vi "ExDataCollectFocus2StripROT.vi"() -> ()   [LabVIEW 2010]
uses:
  Open-Close Hardware/CamHandle.vi
panel:
  out "vert shift time":dbl format="%.2f"
  out "horz shift time":dbl format="%.2f"
  out "Read Out":dbl format="%.2f"
  out "Strip 2":u16[](graph)
  out "Strip":u16[](graph)
  in  "Stop collection":bool
  out "ready to \nstart":bool
  in  "Start collection":bool
  in  "Exposure":dbl min=0.0 step=0.001 format="%.3f"
  out "error out":errorcluster
  in  "error in (no error)":errorcluster
  # "ExDataCollect2StripROT:\nthis example collects data for 2 strips.\nIt also displays the Read Out time, horizontal shift time, and vertical shift time.\nRun this vi and wait for the ready to start to turn green.\nThen hit the start button to collect and display the strips as graphs"
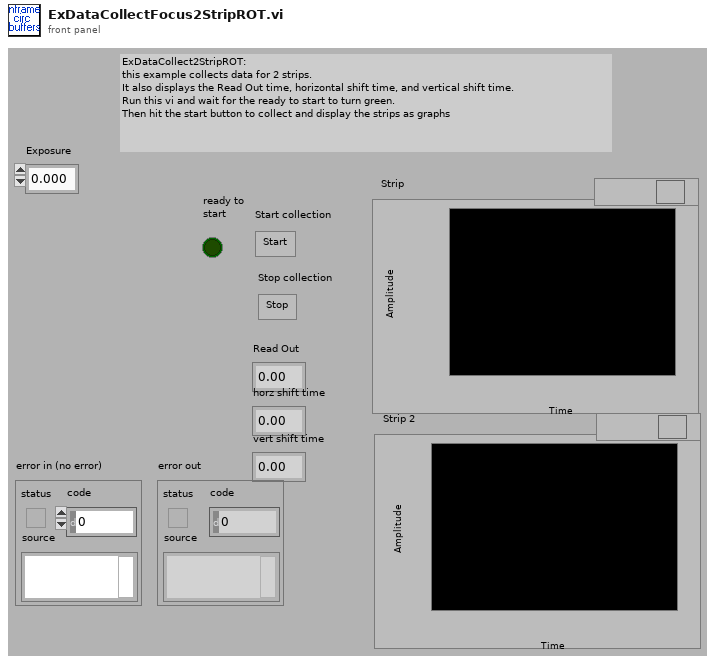
[diagram p1: front panel]
types:
  T1 = cluster{"acquire focus mode":u32, "Exposure":dbl, i32, "Software accumulation":u32}
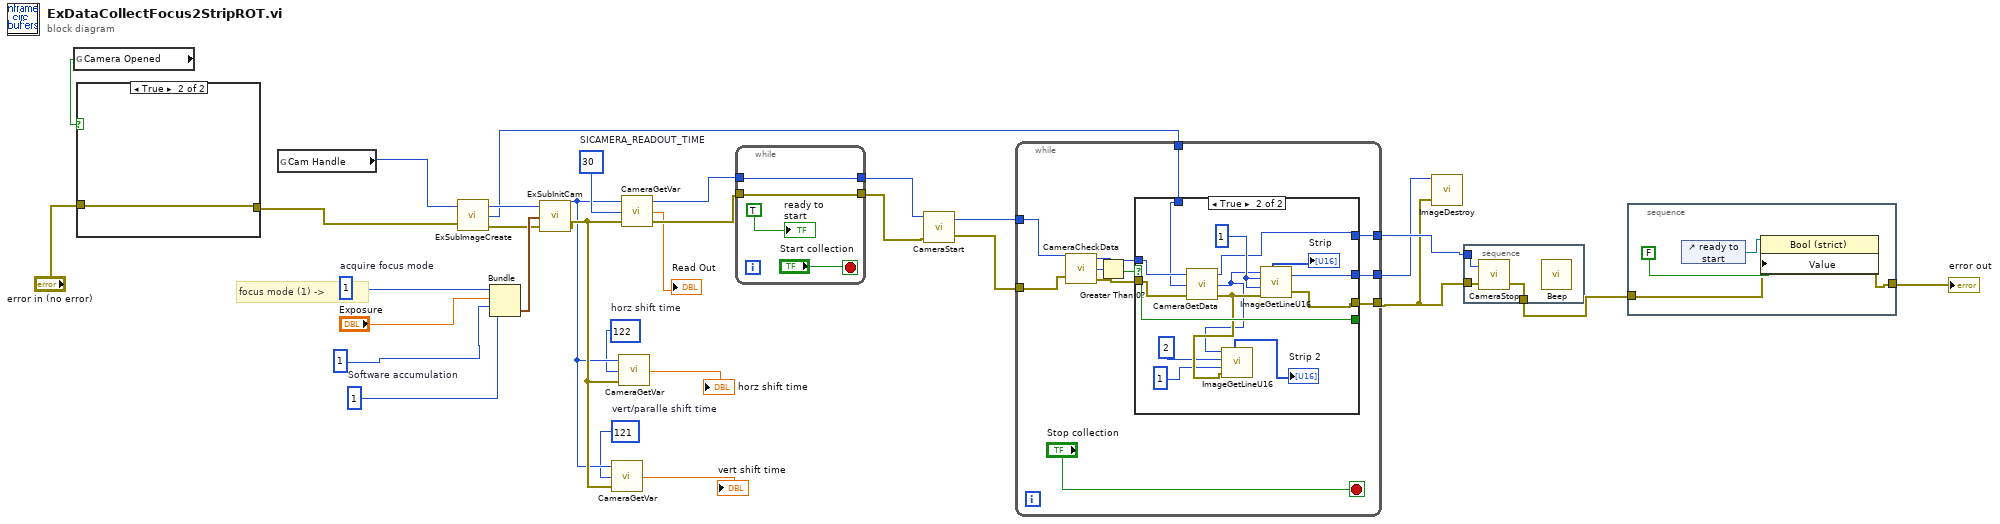
[diagram p0: block diagram]
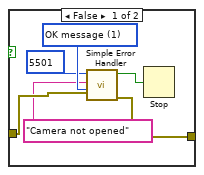
[diagram p3: hidden frame]
diagram:
  w2 = 122  # horz shift time
  w3 = 121  # vert/paralle shift time
  w8 = 30  # SICAMERA_READOUT_TIME
  w29 = u32 1  # acquire focus mode
  w28 = u32 1  # Software accumulation
  # "focus mode (1) ->"
  n1 = global read "CamHandle.vi" "Camera Opened"() -> (w26:bool)
  n2 = case shown="True" w26 {
    tunnel: "error in (no error)" -> [w36 w38]
    tunnel: [w35 w38] -> w18
    frame False {
      w37 = u16 1 items=["no dialog", "OK message", "continue or stop message"] ("type of dialog (OK msg:1)")
      n3 = call <vilib>:"Simple Error Handler.vi"("error code (no error:0)"=5501, "error source (\" \")"="Camera not opened", "type of dialog (OK msg:1)"=w37, "error in (no error)"=w36) -> ("error?"=w33:bool, "error out"=w35:errorcluster)  [unwired: 1 in, 3 out]
      n4 = Stop(stop? (T)=w33) -> ()
    }
    frame True {
    }
  }
  n5 = global read "CamHandle.vi" "Cam Handle"() -> (w20:u32)
  n6 = call "ExSubImageCreate.vi"("Camera Handle"=w20, "error in (no error)"=w18) -> ("Camera Handle"=w19:u32, "Data Handle"=w16:u32, "error out"=w17:errorcluster)
  n7 = Bundle("acquire focus mode"=w29, "Exposure"="Exposure", 1, "Software accumulation"=w28) -> (w30:T1)  [unwired: 1 in]
  n8 = call "ExSubInitCam.vi"("error in (no error)"=w17, "Camera Information"=w30, "Camera Handle"=w19) -> ("error out"=w7:errorcluster, "Camera Handle"=w4:u32)
  n9 = call <userlib>:"CameraGetVar.vi"("error in"=w7, "Parameter ID"=w3, "Camera Handle"=w4) -> ("Value"=→"vert shift time":dbl)  [unwired: 2 out]
  n10 = call <userlib>:"CameraGetVar.vi"("error in"=w7, "Parameter ID"=w2, "Camera Handle"=w4) -> ("Value"=→"horz shift time":dbl)  [unwired: 2 out]
  n11 = call <userlib>:"CameraGetVar.vi"("error in"=w7, "Parameter ID"=w8, "Camera Handle"=w4) -> ("error out"=w11:errorcluster, "Value"=→"Read Out":dbl, "Camera Handle"=w10:u32)
  n12 = while {
    tunnel: w11 -> [w40]
    tunnel: [w40] -> w24
    tunnel: w10 -> [w39]
    tunnel: [w39] -> w23
    stop <- "Start collection" stop-if-true
    "ready to \nstart" <- TRUE
  }
  n13 = call <userlib>:"CameraStart.vi"("error in"=w24, "Camera Handle"=w23) -> ("error out"=w21:errorcluster, "Camera Handle"=w22:u32)
  n14 = while {
    tunnel: w22 -> [w49]
    tunnel: w21 -> [w48]
    tunnel: w16 -> [w46]
    tunnel: [w45] -> w13
    tunnel: [w44] -> w12
    tunnel: [w43] -> w15
    stop <- "Stop collection" stop-if-true
    n15 = call <userlib>:"CameraCheckData.vi"("Camera Handle"=w49, "error in"=w48) -> ("Camera Handle"=w51:u32, "Number Of Frames Available"=w53:i32, "error out"=w50:errorcluster)
    n16 = Greater Than 0?(x=w53) -> (x > 0?=w52:bool)
    n17 = case shown="True" w52 {
      selector: w52 -> [w56 w69]
      tunnel: w51 -> [w54 w71]
      tunnel: w50 -> [w57 w70]
      tunnel: [w56 w69] -> _
      tunnel: [w57 w67] -> w44
      tunnel: w46 -> [w55 w66]
      tunnel: [w55 w64] -> w45
      tunnel: [w54 w63] -> w43
      frame False {
      }
      frame True {
        w65 = 1
        n18 = call <userlib>:"CameraGetData.vi"("error in"=w70, "Data Handle"=w66, "Camera Handle"=w71) -> ("error out"=w62:errorcluster, "Data Handle"=w60:u32, "Camera Handle"=w63:u32)
        n19 = call <userlib>:"ImageGetLineU16.vi"("Data Handle"=w60, "Y Position"=2, "Z Position"=1, "error in"=w62) -> ("Array u16"=→"Strip 2":u16[])  [unwired: 2 out]
        n20 = call <userlib>:"ImageGetLineU16.vi"("Data Handle"=w60, "Y Position"=w65, "Z Position"=w65, "error in"=w62) -> ("Array u16"=→"Strip":u16[], "Data Handle"=w64:u32, "error out"=w67:errorcluster)
      }
    }
  }
  n21 = call <userlib>:"ImageDestroy.vi"("error in"=w12, "Data handle"=w13) -> ()  [unwired: 1 out]
  n22 = stacked-sequence {
    tunnel: w15 -> [w74]
    tunnel: [w73] -> w14
    tunnel: w12 -> [w72]
    frame #0 {
      n23 = call <userlib>:"CameraStop.vi"("error in"=w72, "Camera Handle"=w74) -> ("error out"=w73:errorcluster)  [unwired: 1 out]
      n24 = call <vilib>:"Beep.vi"() -> ()  [unwired: 12 in]
    }
  }
  n25 = stacked-sequence {
    tunnel: [w76] -> w25
    tunnel: w14 -> [w75]
    frame #0 {
      n26 = control-ref of="ready to \nstart"() -> (w78:refnum<vi>)
      n27 = property class="Bool (strict)"(reference=w78, error in=w75, "Value"=FALSE) -> (error out=w76:errorcluster)  [unwired: 1 out]
    }
  }
  "error out" <- w25
